vi "psmc_v2.vi"(0 "F":dbl, 1 "lambda":dbl, 3 "Kp":dbl, 4 "Ki":dbl, 5 "Kd":dbl, 8 "rd":dbl, 9 "T":dbl, 10 "r":dbl, 12 "Reset?":bool) -> (17 "f":dbl)   [LabVIEW 2014]
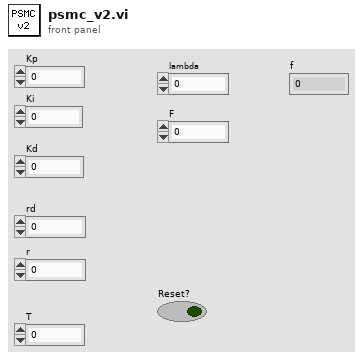
[diagram p1: front panel]
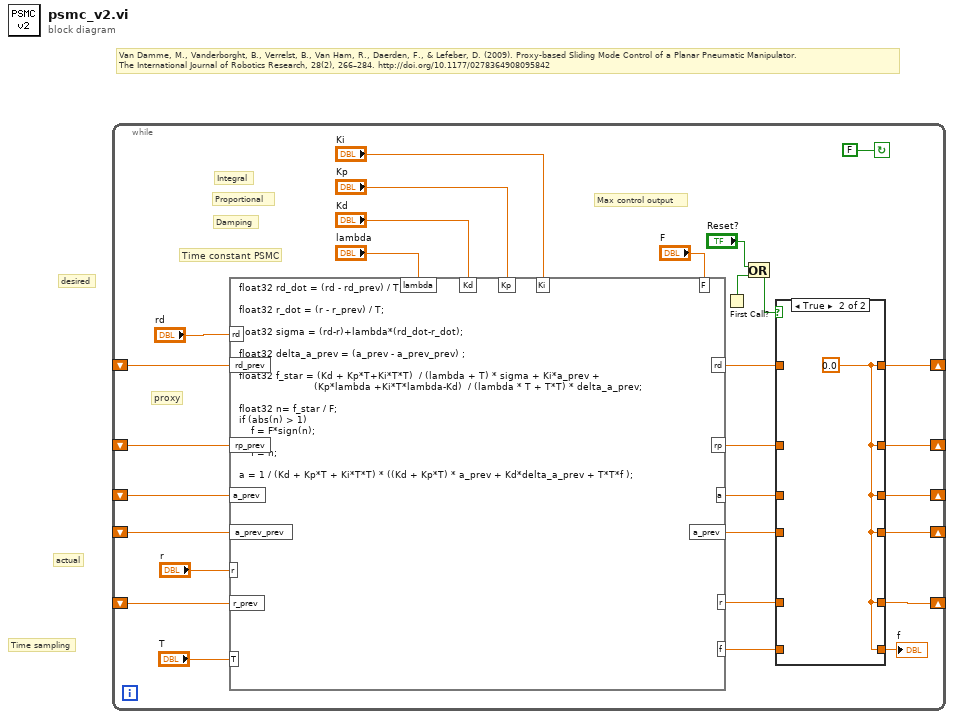
[diagram p0: block diagram]
diagram:
  # "Van Damme, M., Vanderborght, B., Verrelst, B., Van Ham, R., Daerden, F., & Lefeber, D. (2009). Proxy-based Sliding Mode Control of a Planar Pneumatic Manipulator. \nThe International Journal of Robotics Research, 28(2), 266–284. http://doi.org/10.1177/0278364908095842"
  # "Time sampling"
  # "desired"
  # "actual"
  n1 = while {
    shift-right: [w26] -> _
    shift-left: _ -> [w28]
    shift-right: [w25] -> _
    shift-left: _ -> [w27]
    shift-right: [w15] -> _
    shift-left: _ -> [w14]
    shift-right: [w10] -> _
    shift-left: _ -> [w8]
    shift-right: [w6] -> _
    shift-left: _ -> [w7]
    stop <- FALSE continue-if-true
    # "proxy"
    # "Max control output"
    # "Time constant PSMC"
    # "Damping"
    # "Proportional"
    # "Integral"
    n2 = formula code="float32 rd_dot = (rd - rd_prev) / T;\n\nfloat32 r_dot = (r - r_prev) / T;\n\nfloat32 sigma = (rd-r)+lambda*(rd_dot-r_dot);\n\nfloat32 delta_a_prev = (a_prev - a_prev_prev) ;\n\nfloat32 f_star = (Kd + Kp*T+Ki*T*T)  / (lambda + T) * sigma + Ki*a_prev + \n                         (Kp*lambda +Ki*T*lambda-Kd)  / (lambda * T + T*T) * delta_a_prev;\n\nfloat32 n= f_star / F;\nif (abs(n) > 1)\n    f = F*sign(n);\nelse\n    f = n;\n\na = 1 / (Kd + Kp*T + Ki*T*T) * ((Kd + Kp*T) * a_prev + Kd*delta_a_prev + T*T*f );"("T"="T", "rd_prev"=w28, "Kd"="Kd", "Kp"="Kp", "Ki"="Ki", "lambda"="lambda", "rd"="rd", "rp_prev"=w27, "r"="r", "a_prev"=w14, "a_prev_prev"=w8, "F"="F", "r_prev"=w7) -> ("rd"=w24:dbl, "rp"=w23:dbl, "a"=w4:dbl, "f"=w11:dbl, "a_prev"=w9:dbl, "r"=w5:dbl)
    n3 = First Call?() -> (First Call?: T/F=w3:bool)
    n4 = Or(x="Reset?", y=w3) -> (x .or. y?=w2:bool)
    n5 = case shown="True" w2 {
      tunnel: [w35 w36] -> w26
      tunnel: [w34 w36] -> w25
      tunnel: w24 -> [w35 _]
      tunnel: w23 -> [w34 _]
      tunnel: [w33 w36] -> w15
      tunnel: w4 -> [w33 _]
      tunnel: [w32 w36] -> w12
      tunnel: w11 -> [w32 _]
      tunnel: [w31 w36] -> w10
      tunnel: w9 -> [w31 _]
      tunnel: [w30 w36] -> w6
      tunnel: w5 -> [w30 _]
      frame False {
      }
      frame True {
        w36 = 0.0
      }
    }
    "f" <- w12
  }
